vi "Stop Core.vi"(10 "final error code":i32 caption="最终错误代码", 11 "前面板控制 in":refnum<class "前面板控制.lvclass"> caption="操作者输入") -> (3 "前面板控制 out":refnum<class "前面板控制.lvclass"> caption="操作者输出")   [LabVIEW 2015, in "前面板控制.lvlib" / "前面板控制.lvclass"]
doc: "(<B>Filename</B>: Actor Framework.lvlib:Actor.lvclass:Stop Core.vi)\n\nDefines what the actor does before it stops. Use the <B>final error code</B> input to determine whether the actor shut down in response to an error.\n\nBy default, this method does nothing. A descendant class may override it to define behavior, such as shutting down any processes the actor initiated in its override of the Actor Core method."
uses:
  <vilib>/ActorFramework/Actor/Actor.lvclass
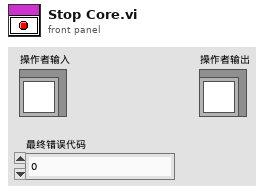
[diagram p1: front panel]
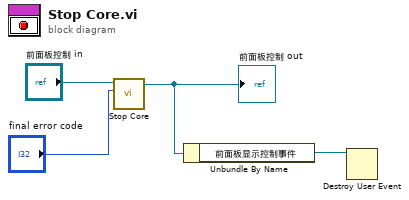
[diagram p0: block diagram]
diagram:
  n1 = call-parent "Stop Core.vi"("final error code"="final error code", "Actor in"="前面板控制 in") -> ("Actor out"=w2:refnum<class "前面板控制.lvclass">)  [unwired: 9 in]
  "前面板控制 out" <- w2
  n2 = Unbundle By Name(w2) -> ("前面板显示控制事件"=w1:refnum<user-event>)
  n3 = Destroy User Event(user event=w1) -> ()  [unwired: 1 in, 1 out]
